vi "Create.vi"(8 "error in (no error)":errorcluster) -> (0 "error out":errorcluster, 3 "DM-DriveForwardDistance.lvclass":refnum<class "DM-DriveForwardDistance.lvclass">)   [LabVIEW 2013, in "DM-DriveForwardDistance.lvclass"]
uses:
  DM-DriveForwardDistance.lvclass
  States/DM-DFD-Starting-State/DM-DFD-Starting-State.lvclass
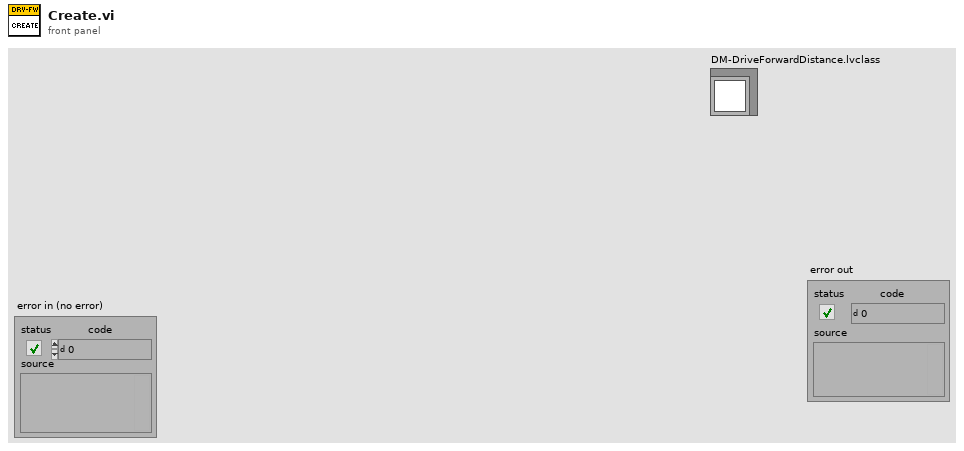
[diagram p1: front panel]
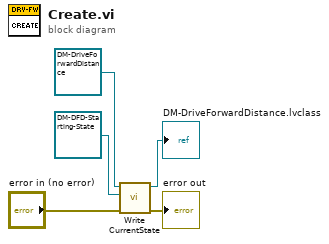
[diagram p0: block diagram]
diagram:
  n1 = call-dynamic "Write CurrentState.vi"("error in (no error)"="error in (no error)", "State.lvclass"=refnum<class "DM-DFD-Starting-State.lvclass"> refnum ("DM-DFD-Starting-State.lvclass"), "Command in"=refnum<class "DM-DriveForwardDistance.lvclass"> refnum ("DM-DriveForwardDistance.lvclass")) -> ("error out"=→"error out":errorcluster, "Command out"=→"DM-DriveForwardDistance.lvclass":refnum<class "DM-DriveForwardDistance.lvclass">)  [unwired: 7 in]
